vi "Read CAN Bus SubVI.vi"(8 "error in (no error)":errorcluster, 9 "seconds since 1Jan1904 in":timestamp, 10 "output cluster in":T1, 11 "Initial Pump Controls":T2 {"Mass Flow SP [kg/h]" min=0.0 max=64.255}) -> (0 "error out":errorcluster, 2 "seconds since 1Jan1904 out":timestamp, 3 "output cluster out":T1)   [LabVIEW 2024, in "Anode.lvlib"]
uses:
  Anode.lvlib
  phlair-busch-can-bus/PumpControls.ctl
  phlair-busch-can-bus/CAN Frame Sessions.ctl
  phlair-busch-can-bus/phlair-busch-can-bus.lvlib
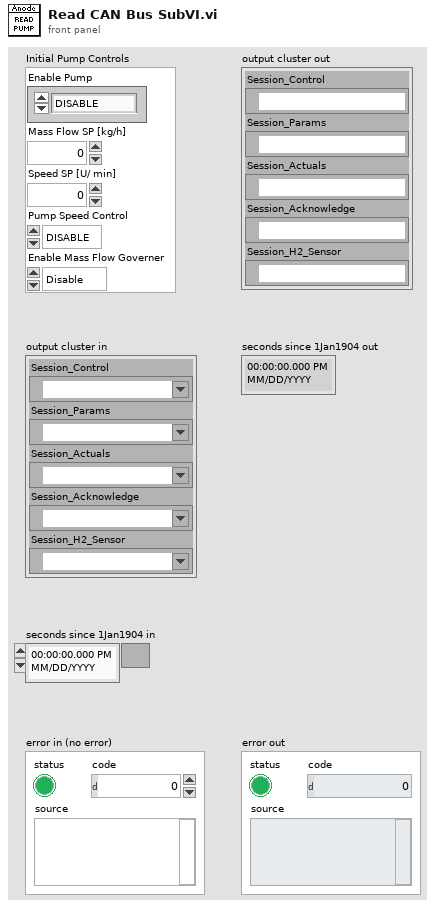
[diagram p1: front panel]
types:
  T1 = typedef "phlair-busch-can-bus.lvlib/CAN Frame Sessions.ctl" = cluster{"Session_Control":refnum<k21>, "Session_Params":refnum<k21>, "Session_Actuals":refnum<k21>, "Session_Acknowledge":refnum<k21>, "Session_H2_Sensor":refnum<k21>}
  T2 = typedef "phlair-busch-can-bus.lvlib/PumpControls.ctl" = cluster{"Enable Pump":enum16{"DISABLE", "ENABLE"}, "Mass Flow SP [kg/h]":dbl, "Speed SP [U/ min]":u16, "Pump Speed Control":enum16{"DISABLE", "ENABLE"}, "Enable Mass Flow Governer":enum8{"Disable", "Enable", "", "NA"}}
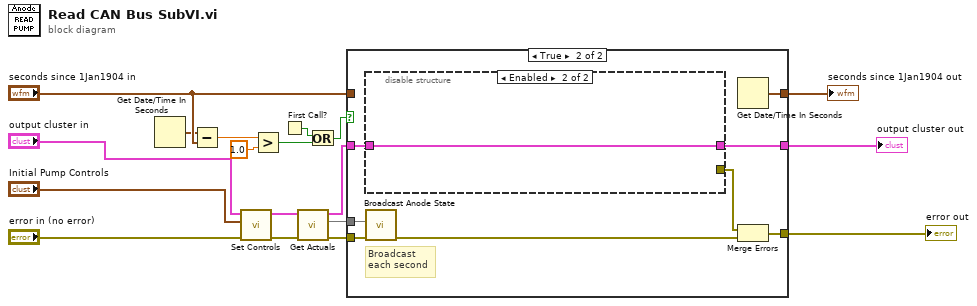
[diagram p0: block diagram]
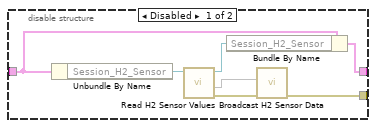
[diagram p3: hidden frame]
diagram:
  n1 = Get Date/Time In Seconds() -> (seconds since 1Jan1904=w11:timestamp)
  n2 = Subtract(x=w11, y="seconds since 1Jan1904 in") -> (x-y=w12:dbl)
  n3 = call "Set Controls.vi"("error in (no error)"="error in (no error)", "Pump Controls"="Initial Pump Controls", "input cluster"="output cluster in") -> ("error out"=w9:errorcluster, "output cluster"=w7:T1)  [unwired: 7 in]
  n4 = Greater?(x=w12, y=1.0) -> (0:w15:bool)
  n5 = First Call?() -> (First Call?: T/F=w17:bool)
  n6 = call "Get Actuals.vi"("error in (no error)"=w9, "input cluster"=w7) -> ("error out"=w5:errorcluster, "Actual Values"=w4:map{string, dbl}, "output cluster"=w3:T1)  [unwired: 7 in]
  n7 = Or(x=w17, y=w15) -> (x .or. y?=w16:bool)
  n8 = case shown="True" w16 {
    tunnel: w4 -> [_ w29]
    tunnel: w5 -> [w21 w28]
    tunnel: [w21 w22] -> w1
    tunnel: [w20 w27] -> w10
    tunnel: "seconds since 1Jan1904 in" -> [w20 _]
    tunnel: w3 -> [w19 w26]
    tunnel: [w19 w25] -> w2
    frame False {
    }
    frame True {
      # "Broadcast\neach second"
      n9 = disable-structure shown="Enabled" {
        disable-tunnel: w26 -> [w35 w37]
        disable-tunnel: [w33 w37] -> w25
        disable-tunnel: [w30 _] -> w24
        frame Disabled {
          n10 = Unbundle By Name(w35) -> ("Session_H2_Sensor"=w34:refnum<k21>)
          n11 = call "Read H2 Sensor Values.vi"("Refnum in"=w34) -> ("error out"=w31:errorcluster, "Data Map"=w36:map{string, dbl}, "Refnum out"=w32:refnum<k21>)  [unwired: 7 in, 1 out]
          n12 = Bundle By Name(cluster=w35, "Session_H2_Sensor"=w32) -> (w33:T1)
          n13 = call "Broadcast H2 Sensor Data.vi"("error in"=w31, "Data Map"=w36) -> ("error out"=w30:errorcluster)  [unwired: 9 in]
        }
        frame Enabled {
        }
      }
      n14 = call "Broadcast Anode State.vi"("error in"=w28, "Anode State Map"=w29) -> ("error out"=w23:errorcluster)  [unwired: 9 in]
      n15 = Get Date/Time In Seconds() -> (seconds since 1Jan1904=w27:timestamp)
      n16 = Merge Errors(w24, w23) -> (w22:errorcluster)
    }
  }
  "seconds since 1Jan1904 out" <- w10
  "output cluster out" <- w2
  "error out" <- w1
